vi "2013FullVi.vi"() -> ()   [LabVIEW 2013]
doc: "Use this template to build a standard state machine design pattern. Each state executes code and determines which state to transition to. Contrast this design pattern with the User Interface Event Handler pattern, in which code executes in response to user actions. Contrast this design pattern also with the Queued Message Handler pattern, in which each message handling code can queue zero or more new messages.\nNote: This template does not contain the most recent programming guidelines recommended by National Instruments. For a complete, project-based implementation of the Standard State Machine pattern, use the Create Project dialog box instead of this template."
uses:
  <vilib>/Math Plots/3D Math Plots/3D Bar/3D Bar Datatype/3D Bar Datatype.lvclass
  <vilib>/Math Plots/3D Math Plots/3D Bar/3D Bar Datatype/Public/Plot Helper (Vector).vi
  <vilib>/express/express arith-compare/Formula/XNode/ExpressFormulaBlockNode.xnode
  <vilib>/University of Leeds/Kinesthesia Toolkit for Microsoft Kinect/_Polymorphic Configure/Event-Depth, Skeleton and Video.vi
  <vilib>/University of Leeds/Kinesthesia Toolkit for Microsoft Kinect/_Polymorphic Read/Read-Depth, Skeleton and Video.vi
  <vilib>/Math Plots/3D Math Plots/3D Bar/3D Bar XCtrl/3D Bar.xctl
  2013Control.ctl
panel:
  in  "Which Joint? (2)":T1(ring)
  out "Joint Coordinates (2)":dbl[](array[numeric])
  out "Joint Coordinates (1)":dbl[](array[numeric])
  in  "Which Joint? (1)":T1(ring)
  out "Base DD":dbl[](array[numeric])
  out "Total DD":dbl[](array[numeric])
  in  "1/2 Twist":dbl[](array[numeric])
  in  "360 Somersault":T2
  in  "1/4 Rotation":dbl[](array[numeric])
  in  "Position":string[](array[combo])
  in  "Skill":string[](array[combo])
  in  "FIG Shorthand":string[](array[string])
  out "Average Jump Time":dbl format="%#.3g"
  out "Standard \nDeviation":dbl format="%#.4g"
  out "Tramp contact":bool
  out "?":refnum<class "3D Plot Datatype.lvclass">[](xcontrol)
  out "Total Air Time":dbl format="%#.3g"
  out "Number of Total Jumps":i32
  out "Number of Official Jumps":i32
  in  "Start Official Jumps":bool
  out "Final Jump Times":dbl[](array[numeric])
  out "Trampoline Time":dbl[](array[numeric])
  out "Air Time":dbl[](array[numeric])
  in  "Stop":bool
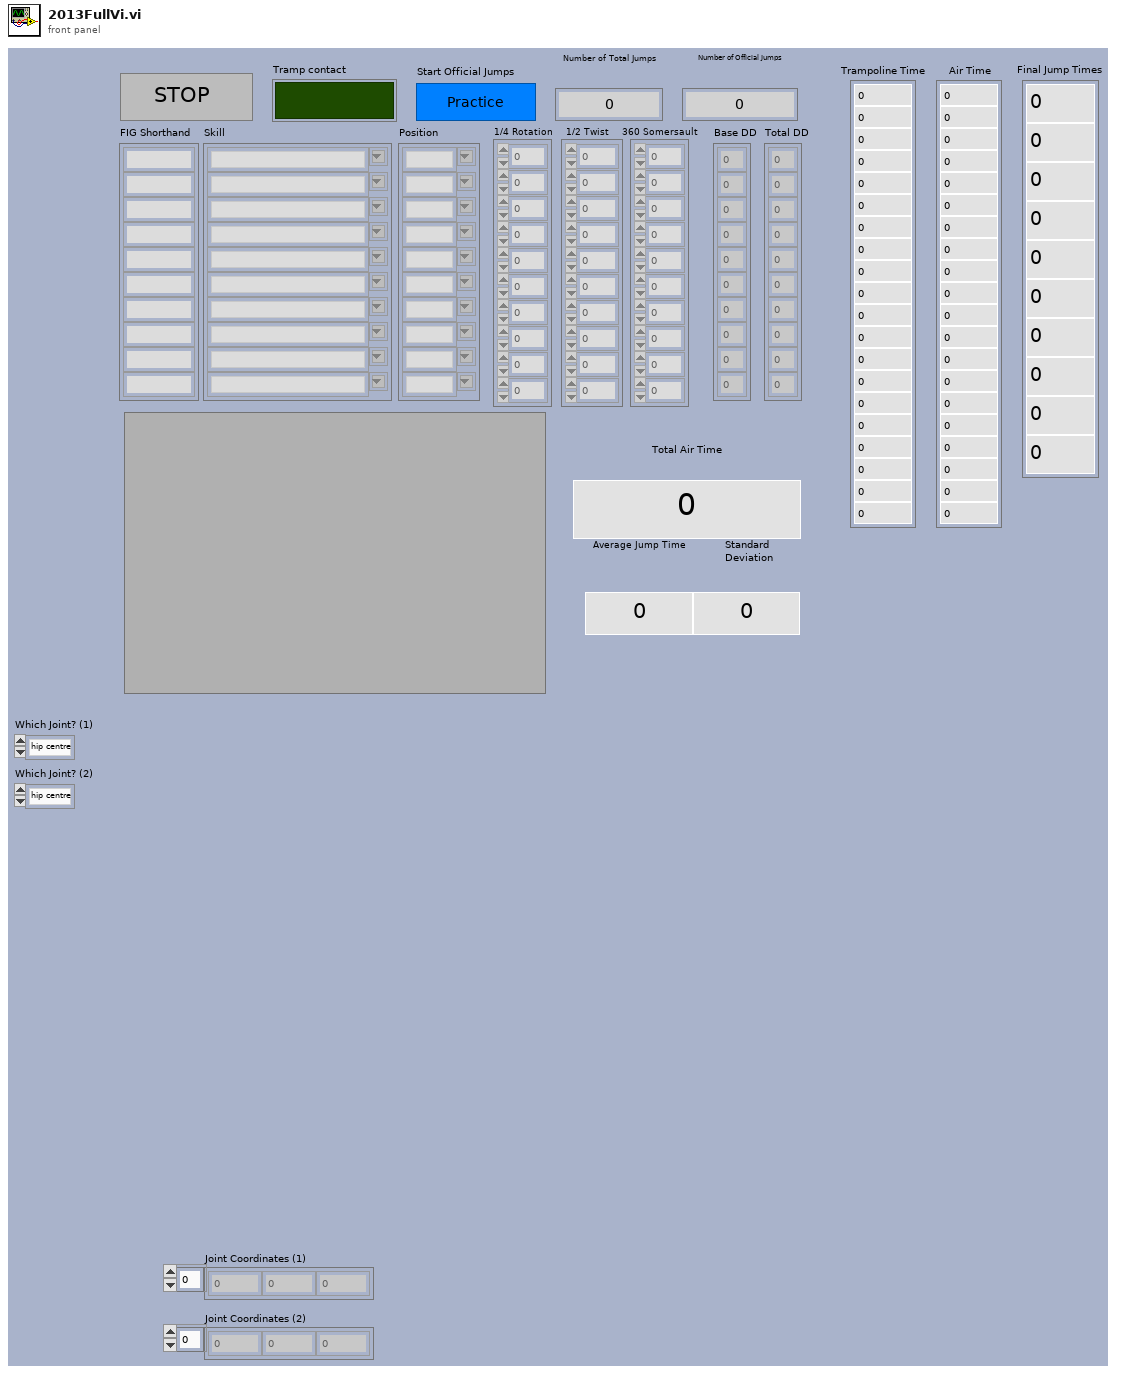
[diagram p1: front panel]
types:
  T1 = enum16{"hip centre", "spine", "shoulder centre", "head", "shoulder left", "elbow left", "wrist left", "hand left", "shoulder right", "elbow right", "wrist right", "hand right", "hip left", "knee left", "ankle left", "foot left", "hip right", "knee right", "ankle right", "foot right"}
  T2 = typedef "2013Control.ctl" = dbl[]
  T3 = cluster{"Start Time":dbl, "Air Time Array ":dbl[], "Tramp Time Array":dbl[], "Number of Jumps  ":i32, "Final Time Array":dbl[], "Number of Final Jumps":i32, "Tramp switch":bool}
  T4 = enum16{"Initialize", "acquire", "analyze", "display", "Stop"}
  T5 = cluster{cluster{"reference out":refnum<k24>, "KinectSensors":refnum<k24>}, "get_Item":refnum<k24>}
  T6 = cluster{"reference out":refnum<k24>, "KinectSensors":refnum<k24>, "SkeletonStream":refnum<k24>, "DepthStream":refnum<k24>, "ColorStream":refnum<k24>, refnum<k24>[], "get_Item":refnum<k24>}
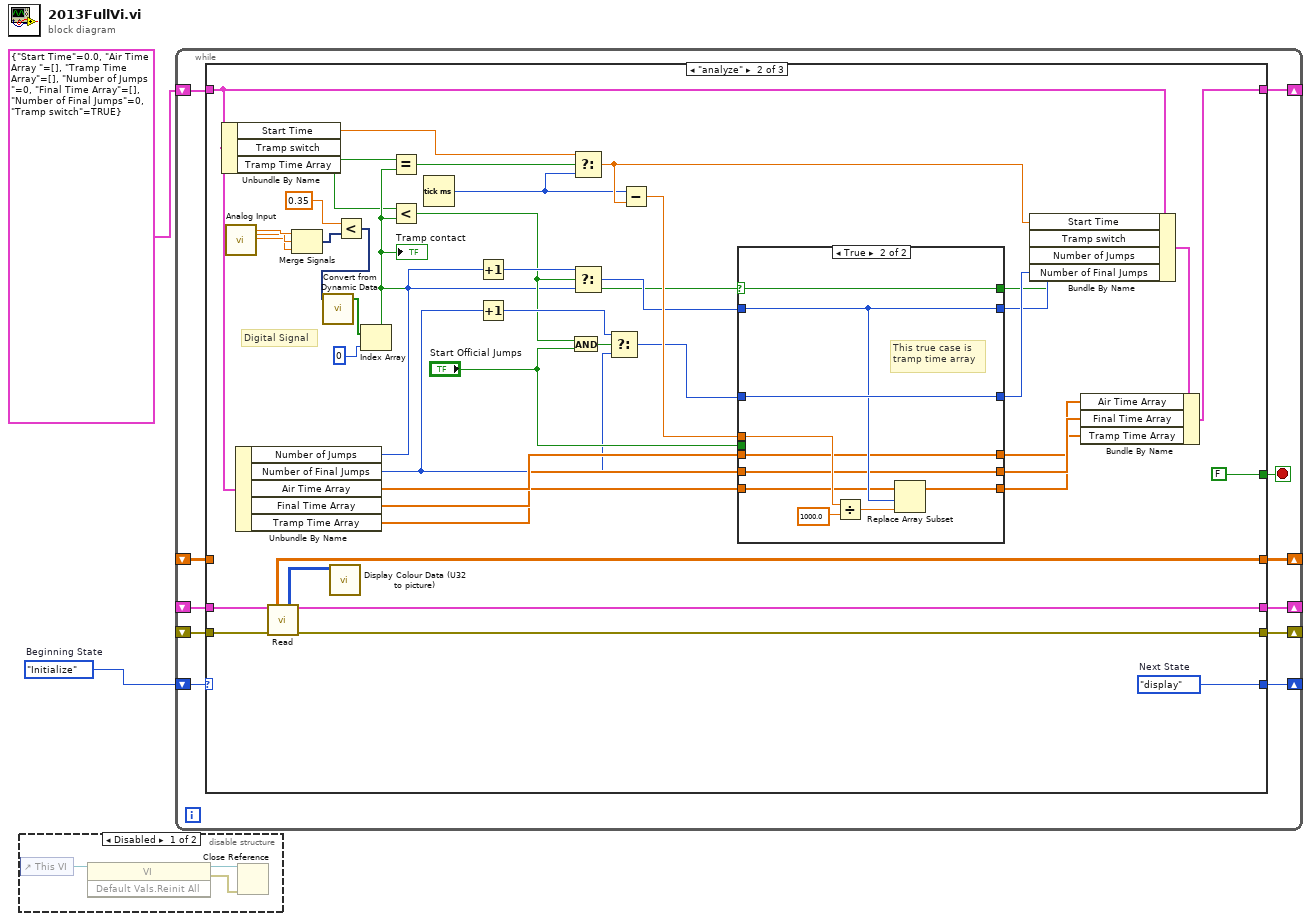
[diagram p0: block diagram]
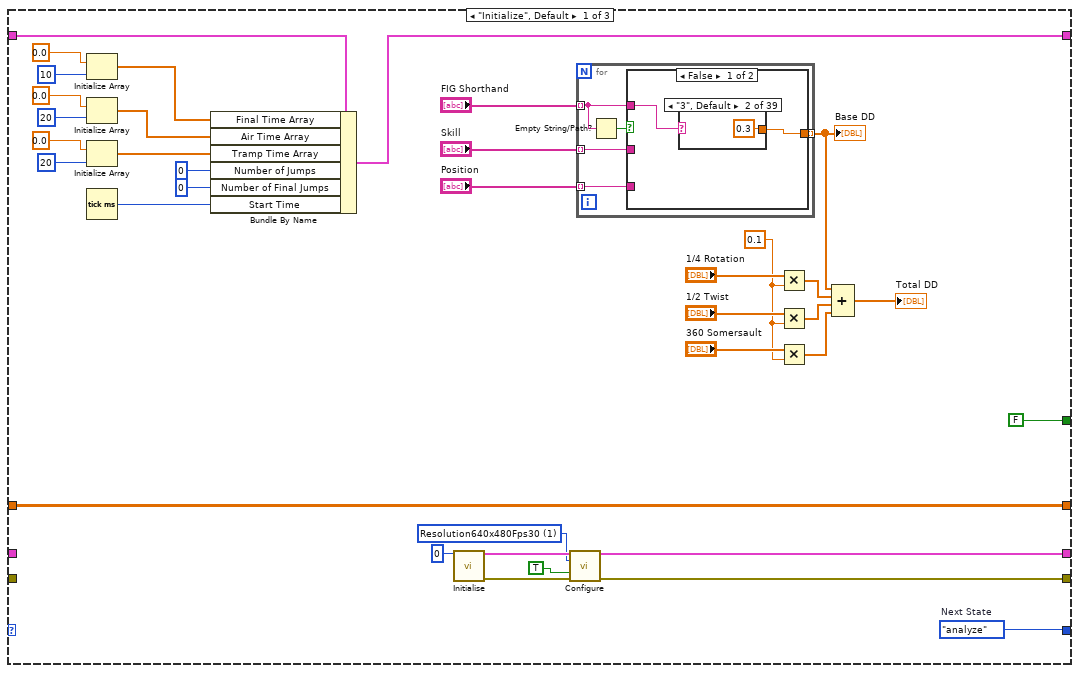
[diagram p3: hidden frame]
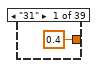
[diagram p4: hidden frame]
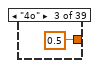
[diagram p5: hidden frame]
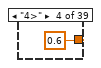
[diagram p6: hidden frame]
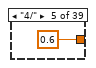
[diagram p7: hidden frame]
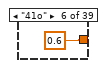
[diagram p8: hidden frame]
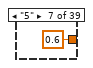
[diagram p9: hidden frame]
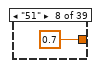
[diagram p10: hidden frame]
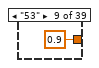
[diagram p11: hidden frame]
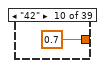
[diagram p12: hidden frame]
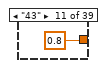
[diagram p13: hidden frame]
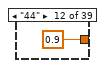
[diagram p14: hidden frame]
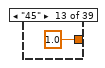
[diagram p15: hidden frame]
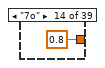
[diagram p16: hidden frame]
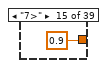
[diagram p17: hidden frame]
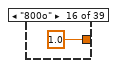
[diagram p18: hidden frame]
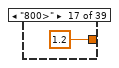
[diagram p19: hidden frame]
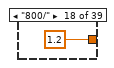
[diagram p20: hidden frame]
diagram:
  w2 = T4."Initialize"  # Beginning State
  n1 = disable-structure shown="Disabled" {
    frame Disabled {
      n2 = control-ref of="This VI"() -> (w5:refnum<vi>)
      n3 = invoke class="VI" method="Default Vals.Reinit All"(reference=w5) -> (reference out=w4:refnum<vi>, error out=w3:errorcluster)  [unwired: 2 in, 1 out]
      n4 = Close Reference(reference=w4, error in (no error)=w3) -> ()  [unwired: 1 out]
    }
    frame Enabled {
    }
  }
  n5 = while {
    shift-right: [w13] -> _
    shift-left: w2 -> [w16]
    shift-right: [w14] -> _
    shift-left: T3 {"Start Time"=0.0, "Air Time Array "=[], "Tramp Time Array"=[], "Number of Jumps  "=0, "Final Time Array"=[], "Number of Final Jumps"=0, "Tramp switch"=TRUE} -> [w15]
    shift-right: [w11] -> _
    shift-left: _ -> [w9]
    shift-right: [w10] -> _
    shift-left: _ -> [w8]
    shift-right: [w7] -> _
    shift-left: _ -> [w6]
    stop <- w12 stop-if-true
    n6 = case shown="\"analyze\"" w16 {
      tunnel: [w52 w230 w290] -> w13
      tunnel: w15 -> [w51 w215 w287]
      tunnel: [w43 w207 w287] -> w14
      tunnel: [FALSE FALSE w288] -> w12
      tunnel: [w19 w195 w262] -> w11
      tunnel: [w18 w196 w264] -> w10
      tunnel: w9 -> [_ w198 w262]
      tunnel: w8 -> [_ w197 w265]
      tunnel: [w17 w194 w263] -> w7
      tunnel: w6 -> [w17 _ w263]
      frame "Initialize", Default {
        w21 = 1 items=["Undefined", "Resolution640x480Fps30", "Resolution320x240Fps30", "Resolution80x60Fps30"] ("Depth Stream Format")
        w28 = 0.1
        w52 = T4."analyze"  # Next State
        n7 = Initialize Array(0.0 ("element"), 10 ("dimension size")) -> (w40:dbl[])
        n8 = Initialize Array(0.0 ("element"), 20 ("dimension size")) -> (w47:dbl[])
        n9 = Initialize Array(0.0 ("element"), 20 ("dimension size")) -> (w44:dbl[])
        n10 = Tick Count (ms)() -> (millisecond timer value=w37:u32)
        n11 = Bundle By Name(cluster=w51, "Final Time Array"=w40, "Air Time Array"=w47, "Tramp Time Array"=w44, "Number of Jumps"=0 ("Tramp release"), "Number of Final Jumps"=0, "Start Time"=w37) -> (w43:T3)
        n12 = call <vilib>:"Initialise.vi"("Kinect Number"=0) -> ("Kinect References out"=w24:T5, "error out"=w23:errorcluster)  [unwired: 13 in]
        n13 = call-poly <vilib>:"Configure.vi"("Kinect References in"=w24, "Depth Stream Format"=w21, "Skeleton Smoothing"=TRUE, "error in"=w23) -> ("Kinect References out"=w19:T6, "error out"=w18:errorcluster)  [unwired: 10 in]
        n14 = for {
          tunnel: "FIG Shorthand" -> [w55] mode=indexing
          tunnel: [w57] -> w29 mode=indexing
          tunnel: "Skill" -> [w54] mode=indexing
          tunnel: "Position" -> [w53] mode=indexing
          n15 = Empty String/Path?(string/path=w55) -> (empty?=w56:bool)
          n16 = case shown="False" w56 {
            tunnel: w55 -> [w59 _]
            tunnel: [w58 w99] -> w57
            tunnel: w54 -> [_ w101]
            tunnel: w53 -> [_ w100]
            frame False {
              n17 = case shown="\"3\", Default" w59 {
                tunnel: [0.4 0.3 0.5 0.6 0.6 0.6 0.6 0.7 0.9 0.7 0.8 0.9 1.0 0.8 0.9 1.0 1.2 1.2 1.1 1.1 1.3 1.3 1.5 1.3 1.5 1.7 2.0 0.6 0.7 0.8 1.1 1.2 1.4 1.4 1.6 1.2 1.4 1.4 1.6] -> w58
                frame "31" {
                }
                frame "3", Default {
                }
                frame "4o" {
                }
                frame "4>" {
                }
                frame "4/" {
                }
                frame "41o" {
                }
                frame "5" {
                }
                frame "51" {
                }
                frame "53" {
                }
                frame "42" {
                }
                frame "43" {
                }
                frame "44" {
                }
                frame "45" {
                }
                frame "7o" {
                }
                frame "7>" {
                }
                frame "800o" {
                }
                frame "800>" {
                }
                frame "800/" {
                }
                frame "810o" {
                }
                frame "801o" {
                }
                frame "801>" {
                }
                frame "821o" {
                }
                frame "821/" {
                }
                frame "803o" {
                }
                frame "803>" {
                }
                frame "12001o" {
                }
                frame "12001>" {
                }
                frame "5o" {
                }
                frame "5>" {
                }
                frame "52" {
                }
                frame "46" {
                }
                frame "802o" {
                }
                frame "802/" {
                }
                frame "822o" {
                }
                frame "822/" {
                }
                frame "811o" {
                }
                frame "811>" {
                }
                frame "813o" {
                }
                frame "813>" {
                }
              }
            }
            frame True {
              n18 = case shown="\"Full Out\"" w101 {
                tunnel: w100 -> [_ _ w104 w109 _ _ _ _ _ _ _ w121 w125 _ w131 w135 w139 w143 _ w149 w154 _ _ _ _ w163 w166 w171 w175 w179 w184]
                tunnel: [0.3 0.4 w105 w110 0.6 0.7 0.9 0.7 0.8 0.9 1.0 w122 w126 1.1 w132 w136 w140 w144 0.3 w148 w153 0.7 0.8 0.9 1.1 w162 w167 w172 w176 w180 w183] -> w99
                frame "3/4 Front", Default {
                }
                frame "Arabian 3/4 Front" {
                }
                frame "Front" {
                  n19 = case shown="\"Straight\"" w104 {
                    tunnel: [0.6 0.6 0.5] -> w105
                    frame "Straight" {
                    }
                    frame "Pike" {
                    }
                    frame "Tuck", Default {
                    }
                  }
                }
                frame "Barani" {
                  n20 = case shown="\"Straight\"" w109 {
                    tunnel: [0.6 0.6 0.6] -> w110
                    frame "Straight" {
                    }
                    frame "Pike" {
                    }
                    frame "Tuck", Default {
                    }
                  }
                }
                frame "Ballout" {
                }
                frame "Barani Ballout" {
                }
                frame "Rudy Ballout" {
                }
                frame "Front Full" {
                }
                frame "Rudi" {
                }
                frame "Front Double Full" {
                }
                frame "Randi" {
                }
                frame "1 3/4 Front" {
                  n21 = case shown="\"Tuck\", Default" w121 {
                    tunnel: [0.9 0.8] -> w122
                    frame "Pike" {
                    }
                    frame "Tuck", Default {
                    }
                  }
                }
                frame "Double Front" {
                  n22 = case shown="\"Pike\"" w125 {
                    tunnel: [1.2 1.2 1.0] -> w126
                    frame "Straight" {
                    }
                    frame "Pike" {
                    }
                    frame "Tuck", Default {
                    }
                  }
                }
                frame "Half In Back Out" {
                }
                frame "Half Out" {
                  n23 = case shown="\"Tuck\", Default" w131 {
                    tunnel: [1.3 1.1] -> w132
                    frame "Pike" {
                    }
                    frame "Tuck", Default {
                    }
                  }
                }
                frame "Full Barani" {
                  n24 = case shown="\"Tuck\", Default" w135 {
                    tunnel: [1.5 1.1] -> w136
                    frame "Straight" {
                    }
                    frame "Tuck", Default {
                    }
                  }
                }
                frame "Rudi Out" {
                  n25 = case shown="\"Tuck\", Default" w139 {
                    tunnel: [1.5 1.3] -> w140
                    frame "Pike" {
                    }
                    frame "Tuck", Default {
                    }
                  }
                }
                frame "Triffus" {
                  n26 = case shown="\"Tuck\", Default" w143 {
                    tunnel: [2.0 1.7] -> w144
                    frame "Pike" {
                    }
                    frame "Tuck", Default {
                    }
                  }
                }
                frame "3/4 Back" {
                }
                frame "Back" {
                  n27 = case shown="\"Straight\"" w149 {
                    tunnel: [0.6 0.6 0.5] -> w148
                    frame "Pike" {
                    }
                    frame "Straight" {
                    }
                    frame "Tuck", Default {
                    }
                  }
                }
                frame "Cody" {
                  n28 = case shown="\"Straight\"" w154 {
                    tunnel: [0.7 0.8 0.6] -> w153
                    frame "Pike" {
                    }
                    frame "Straight" {
                    }
                    frame "Tuck", Default {
                    }
                  }
                }
                frame "Back Full" {
                }
                frame "Back 1 1/2 Full" {
                }
                frame "Back Double Full" {
                }
                frame "Back Triple Full" {
                }
                frame "1 3/4 Back" {
                  n29 = case shown="\"Tuck\", Default" w163 {
                    tunnel: [0.9 0.8] -> w162
                    frame "Pike" {
                    }
                    frame "Tuck", Default {
                    }
                  }
                }
                frame "Double Back" {
                  n30 = case shown="\"Tuck\", Default" w166 {
                    tunnel: [1.2 1.2 1.0] -> w167
                    frame "Straight" {
                    }
                    frame "Pike" {
                    }
                    frame "Tuck", Default {
                    }
                  }
                }
                frame "Full Out" {
                  n31 = case shown="\"Tuck\", Default" w171 {
                    tunnel: [1.4 1.2] -> w172
                    frame "Straight" {
                    }
                    frame "Tuck", Default {
                    }
                  }
                }
                frame "Full Full" {
                  n32 = case shown="\"Tuck\", Default" w175 {
                    tunnel: [1.6 1.4] -> w176
                    frame "Straight" {
                    }
                    frame "Tuck", Default {
                    }
                  }
                }
                frame "Half Half" {
                  n33 = case shown="\"Tuck\", Default" w179 {
                    tunnel: [1.4 1.2] -> w180
                    frame "Pike" {
                    }
                    frame "Tuck", Default {
                    }
                  }
                }
                frame "Half Rudi" {
                  n34 = case shown="\"Tuck\", Default" w184 {
                    tunnel: [1.6 1.4] -> w183
                    frame "Pike" {
                    }
                    frame "Tuck", Default {
                    }
                  }
                }
              }
            }
          }
        }
        "Base DD" <- w29
        n35 = Multiply(x="1/4 Rotation", y=w28) -> (x*y=w33:dbl[])
        n36 = Multiply(x="1/2 Twist", y=w28) -> (x*y=w32:dbl[])
        n37 = Multiply(x="360 Somersault", y=w28) -> (x*y=w31:T2)
        n38 = Compound Arithmetic op=ADD(w29, w33, w32, w31) -> (→"Total DD":T2)
      }
      frame "analyze" {
        w230 = T4."display"  # Next State
        # "Digital Signal"
        n39 = Unbundle By Name(w215) -> ("Start Time"=w205:dbl, "Tramp switch"=w200:bool)  [unwired: 1 out]
        n40 = call "Analog Input"() -> ("A/AI1 (Pin 5)"=w193:dbl, "A/AI2 (Pin 7)"=w192:dbl, "A/AI3 (Pin 9)"=w191:dbl)  [unwired: 24 in, 1 out]
        n41 = Unbundle By Name(w215) -> ("Number of Jumps"=w203:i32, "Number of Final Jumps"=w204:i32, "Air Time Array"=w220:dbl[], "Final Time Array"=w219:dbl[], "Tramp Time Array"=w213:dbl[])
        n42 = call-poly <vilib>:"Read.vi"("Kinect References in"=w198, "error in (no error)"=w197) -> ("Primary Skeleton Array"=w194:dbl[][], "Colour output array (U24, RGB)"=w199:u32[][], "Kinect References out"=w195:T6, "error out"=w196:errorcluster)  [unwired: 8 in, 2 out]
        n43 = Merge Signals(w193, w192, w191) -> (w189:dynamicdata)
        n44 = call <vilib>:"Display Colour Data (U32 to picture).vi"("Colour output array (U24, RGB)"=w199) -> ()  [unwired: 10 in, 1 out]
        n45 = Less?(x=0.35, y=w189) -> (x < y?=w188:dynamicdata)
        n46 = call "Convert from Dynamic Data"("Dynamic Data Type"=w188) -> ("Array"=w187:bool[])  [unwired: 3 in]
        n47 = Index Array(array=w187, index=0) -> (element=w201:bool)
        "Tramp contact" <- w201
        n48 = Equal?(x=w200, y=w201) -> (x = y?=w227:bool)
        n49 = Less?(x=w200, y=w201) -> (x < y?=w217:bool)
        n50 = Tick Count (ms)() -> (millisecond timer value=w206:u32)
        n51 = Increment(x=w203) -> (x+1=w228:i32)
        n52 = Increment(x=w204) -> (x+1=w224:i32)
        n53 = And(x=w217, y="Start Official Jumps") -> (x .and. y?=w222:bool)
        n54 = Select(t=w205, s=w227, f=w206) -> (s? t:f=w218:dbl)
        n55 = Select(t=w228, s=w217, f=w203) -> (s? t:f=w221:i32)
        n56 = Select(t=w224, s=w222, f=w204) -> (s? t:f=w223:i32)
        n57 = Subtract(x=w206, y=w218) -> (x-y=w226:dbl)
        n58 = case shown="True" w201 {
          selector: w201 -> [w231 w254]
          tunnel: [w232 w257] -> w209
          tunnel: [w243 w252] -> w211
          tunnel: w219 -> [w234 w253]
          tunnel: w221 -> [w233 w256]
          tunnel: w226 -> [w236 w259]
          tunnel: w220 -> [w235 w252]
          tunnel: [w242 w253] -> w212
          tunnel: w223 -> [w241 w261]
          tunnel: [w240 w261] -> w225
          tunnel: "Start Official Jumps" -> [w239 _]
          tunnel: [w233 w256] -> w214
          tunnel: w213 -> [w232 w255]
          tunnel: [w231 w254] -> w210
          frame False {
            n59 = case shown="True" w239 {
              tunnel: w236 -> [_ w247]
              tunnel: [w245 w250] -> w242
              tunnel: w234 -> [w245 w251]
              tunnel: w241 -> [w244 w246]
              tunnel: [w244 w246] -> w240
              frame False {
              }
              frame True {
                n60 = Divide(x=w247, y=1000.0) -> (x/y=w248:dbl)
                n61 = Replace Array Subset(array=w251, new element=w248, index=w246) -> (w250:dbl[])
              }
            }
            n62 = Divide(x=w236, y=1000.0) -> (x/y=w237:dbl)
            n63 = Replace Array Subset(array=w235, new element=w237, index=w233) -> (w243:dbl[])
          }
          frame True {
            # "This true case is tramp time array"
            n64 = Divide(x=w259, y=1000.0) -> (x/y=w258:dbl)
            n65 = Replace Array Subset(array=w255, new element=w258, index=w256) -> (w257:dbl[])
          }
        }
        n66 = Bundle By Name(cluster=w215, "Start Time"=w218, "Tramp switch"=w210, "Number of Jumps"=w214, "Number of Final Jumps"=w225) -> (w208:T3)
        n67 = Bundle By Name(cluster=w208, "Air Time Array"=w211, "Final Time Array"=w212, "Tramp Time Array"=w209) -> (w207:T3)
      }
      frame "display" {
        w290 = T4."analyze"  # Next State
        n68 = Unbundle By Name(w287) -> ("Air Time Array"=→"Air Time":dbl[], "Tramp Time Array"=→"Trampoline Time":dbl[], "Final Time Array"=w278:dbl[])
        "Final Jump Times" <- w278
        n69 = call <vilib>:"Joint Coordinates.vi"("error in (no error)"=w265, "Joint 1"="Which Joint? (1)", "Array of Joint Positions"=w263) -> ("error out"=w266:errorcluster, "Joint Coordinates"=→"Joint Coordinates (1)":dbl[])  [unwired: 7 in]
        n70 = Add Array Elements(numeric array=w278) -> (sum=w277:dbl)
        "Total Air Time" <- w277
        n71 = Divide(x=w277, y=10.0) -> (x/y=w271:dbl)
        "Average Jump Time" <- w271
        n72 = call-poly <vilib>:"Plot Helper.vi"("z vector"=w278, "y vector"=sgl[] [1.0, 2.0, 3.0, 4.0, 5.0, 6.0, 7.0, 8.0, 9.0, 10.0]) -> ("3D Plot lvclass Array out"=→"?":refnum<class "3D Plot Datatype.lvclass">[])  [unwired: 1 in, 8 out]
        n73 = Unbundle By Name(w287) -> ("Number of Jumps"=→"Number of Total Jumps":i32, "Number of Final Jumps"=w285:i32)
        "Number of Official Jumps" <- w285
        n74 = call <vilib>:"Joint Coordinates.vi"("error in (no error)"=w266, "Joint 1"="Which Joint? (2)", "Array of Joint Positions"=w263) -> ("error out"=w264:errorcluster, "Joint Coordinates"=→"Joint Coordinates (2)":dbl[])  [unwired: 7 in]
        n75 = for {
          N: 10 -> [_]
          tunnel: w278 -> [w292] mode=indexing
          tunnel: w271 -> [w293]
          tunnel: [w291] -> w275 mode=indexing
          n76 = xnode "Formula"("Jump Time"=w292, "Average"=w293) -> ("Result"=w291:dbl)  [unwired: 1 in, 1 out]
        }
        n77 = Add Array Elements(numeric array=w275) -> (sum=w273:dbl)
        n78 = Square Root(x=w273) -> (sqrt(x)=→"Standard \nDeviation":dbl)
        n79 = Greater Or Equal?(x=w285, y=10) -> (x >= y?=w280:bool)
        n80 = Or(x=w280, y="Stop") -> (x .or. y?=w288:bool)
      }
    }
  }
